vi "SCAR TRIAL WITH TCP SERVER.vi"(7 "Enum":enum16{"INIT", "READ", "WRITE", "CLOSE"}(ring), 8 "error in":errorcluster, 11 "String":string="CLOSE") -> (0 "error out":errorcluster, 2 "data out":string)   [LabVIEW 2023]
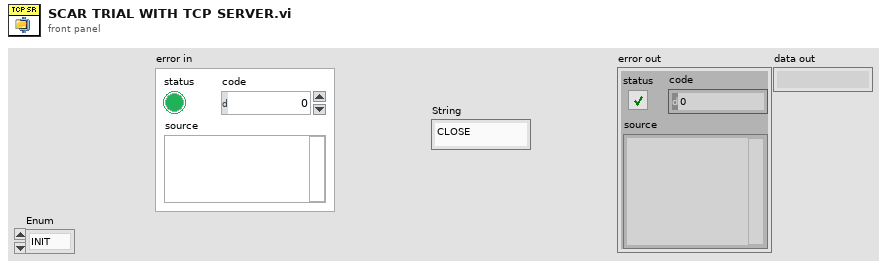
[diagram p1: front panel]
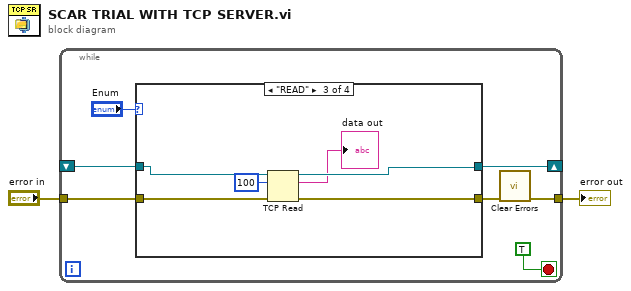
[diagram p0: block diagram]
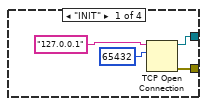
[diagram p2: hidden frame]
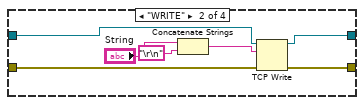
[diagram p3: hidden frame]
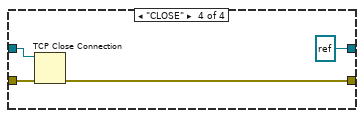
[diagram p4: hidden frame]
diagram:
  n1 = while {
    tunnel: [w3] -> w1
    shift-right: [w7] -> _
    shift-left: _ -> [w5]
    tunnel: "error in" -> [w4]
    stop <- TRUE ("stop 2") stop-if-true
    n2 = case shown="\"READ\"" "Enum" {
      tunnel: [w11 w19 w23 refnum<k5> refnum ("connection ID")] -> w7
      tunnel: [w10 w17 w24 w28] -> w6
      tunnel: w5 -> [_ w20 w25 w29]
      tunnel: w4 -> [_ w18 w26 w30]
      frame "INIT" {
        n3 = TCP Open Connection(address="127.0.0.1", remote port or service name=u16 65432) -> (connection ID=w11:refnum<k5>, error out=w10:errorcluster)  [unwired: 3 in]
      }
      frame "WRITE" {
        n4 = Concatenate Strings("String", "\r\n") -> (w14:string)
        n5 = TCP Write(connection ID=w20, data in=w14, error in (no error)=w18) -> (connection ID out=w19:refnum<k5>, error out=w17:errorcluster)  [unwired: 1 in, 1 out]
      }
      frame "READ" {
        n6 = TCP Read(connection ID=w25, bytes to read=100, error in (no error)=w26) -> (connection ID out=w23:refnum<k5>, data out=→"data out":string, error out=w24:errorcluster)  [unwired: 2 in]
      }
      frame "CLOSE" {
        n7 = TCP Close Connection(connection ID=w29, error in (no error)=w30) -> (error out=w28:errorcluster)  [unwired: 1 in, 1 out]
      }
    }
    n8 = call <vilib>:"Clear Errors.vi"("error in (no error)"=w6) -> ("error out"=w3:errorcluster)  [unwired: 5 in, 1 out]
  }
  "error out" <- w1
